vi "pipx40 Close.vi"(8 "error in (no error)":errorcluster, 11 "instrument handle":refnum<visa-resource-name>) -> (0 "error out":errorcluster, 3 "status":i32)   [LabVIEW 2011]
doc: "Terminates the software connection to the card and deallocates system resources associated with the card.\n\nNOTE: the card must be re-initialized to use it again."
uses:
  pipx40_32.dll
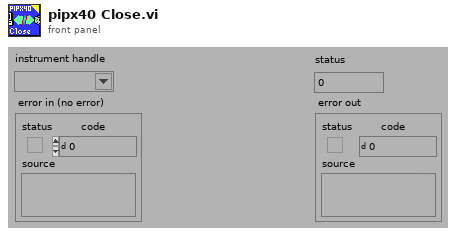
[diagram p1: front panel]
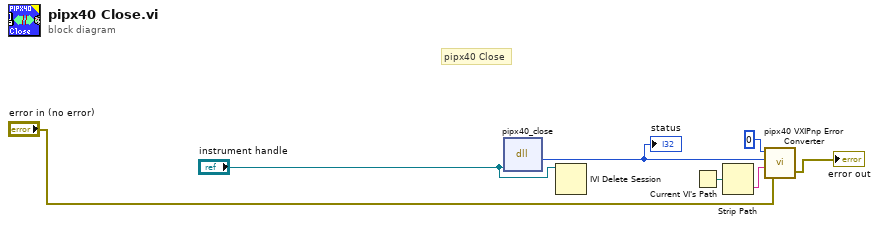
[diagram p0: block diagram]
diagram:
  # "pipx40 Close"
  n1 = dll-call lib="pipx40_32.dll" fn="pipx40_close" label="pipx40Close"("instrument handle"="instrument handle") -> ("status"=w1:i32)  [unwired: 4 in, 2 out]
  "status" <- w1
  n2 = IVI Delete Session(11:"instrument handle") -> ()
  n3 = Current VI's Path() -> (path=w7:path)
  n4 = Strip Path(path=w7) -> (name=w6:string)  [unwired: 1 out]
  n5 = call "pipx40 VXIPnp Error Converter.vi"("error in (no error)"="error in (no error)", "name of VI (\"\")"=w6, "VXIPnp error code (0)"=w1, "instrument handle"=i8 0) -> ("error out"=→"error out":errorcluster)  [unwired: 1 out]
